vi "DeCoF wait for prompt.vi"(0 "Connection ID in":T1, 2 "time out (ms)":i32=1000, 3 "error in (no error)":errorcluster) -> (4 "complete answer":string, 5 "Conncection ID out":T1, 6 "answer string":string, 7 "timed out?":bool, 8 "error out":errorcluster)   [LabVIEW 2013]
doc: "This VI collects the input from the remote connection until the prompt string is found or the timeout expires.\nThe answer string contains the complete collected string minus the prompt, if found."
uses:
  DeCoF connection.ctl
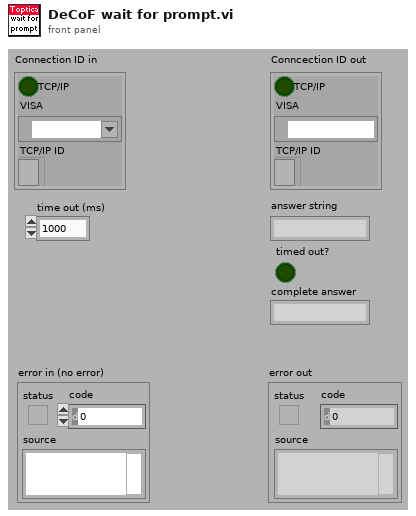
[diagram p1: front panel]
types:
  T1 = typedef "DeCoF connection.ctl" = cluster{"TCP/IP":bool, "VISA":refnum<visa-resource-name>, "TCP/IP ID":refnum<k5>}
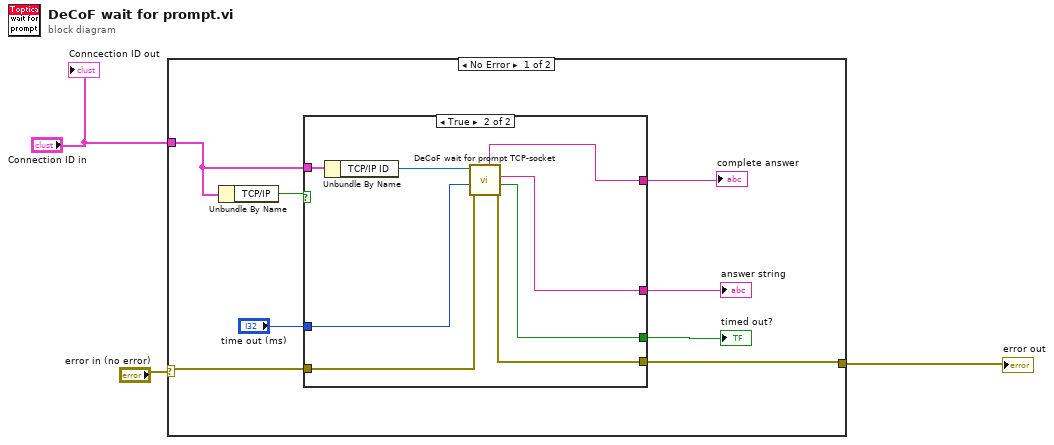
[diagram p0: block diagram]
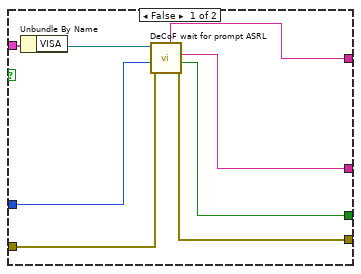
[diagram p2: hidden frame]
diagram:
  n1 = case shown="No Error" "error in (no error)" {
    selector: "error in (no error)" -> [w11 w28]
    tunnel: [w8 w28] -> w2
    tunnel: "Connection ID in" -> [w6 _]
    frame No Error {
      n2 = Unbundle By Name(w6) -> ("TCP/IP"=w5:bool)
      n3 = case shown="True" w5 {
        tunnel: w6 -> [w14 w22]
        tunnel: w11 -> [w18 w26]
        tunnel: "time out (ms)" -> [w19 w27]
        tunnel: [w17 w25] -> w8
        tunnel: [w16 w24] -> w9
        tunnel: [w15 w23] -> w4
        tunnel: [w12 w20] -> w7
        frame False {
          n4 = Unbundle By Name(w14) -> ("VISA"=w13:refnum<visa-resource-name>)
          n5 = call "DeCoF wait for prompt ASRL.vi"("error in (no error)"=w18, "time out (ms)"=w19, "VISA resource name"=w13) -> ("error out"=w17:errorcluster, "timed out?"=w16:bool, "answer string"=w15:string, "complete answer"=w12:string)  [unwired: 2 in, 1 out]
        }
        frame True {
          n6 = Unbundle By Name(w22) -> ("TCP/IP ID"=w21:refnum<k5>)
          n7 = call "DeCoF wait for prompt TCP-socket.vi"("error in (no error)"=w26, "time out (ms)"=w27, "Connection ID"=w21) -> ("error out"=w25:errorcluster, "timed out?"=w24:bool, "answer string"=w23:string, "complete answer"=w20:string)  [unwired: 2 in, 1 out]
        }
      }
      "timed out?" <- w9
      "answer string" <- w4
      "complete answer" <- w7
    }
    frame Error {
    }
  }
  "error out" <- w2
  "Conncection ID out" <- "Connection ID in"
